vi "Event_Structure.vi"() -> ()   [LabVIEW 2022 SP3]
panel:
  out "Numeric":i32
  out "String":string
  in  "Close Button":bool
  in  "Open Button":bool
  out "Boolean":bool
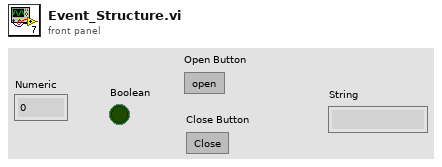
[diagram p1: front panel]
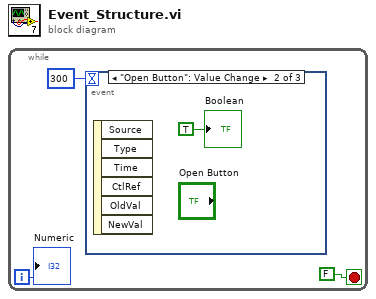
[diagram p0: block diagram]
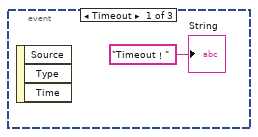
[diagram p2: hidden frame]
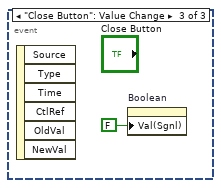
[diagram p3: hidden frame]
diagram:
  n1 = while {
    i -> [w1]
    stop <- FALSE stop-if-true
    n2 = event shown="[1] \"Open Button\": Value Change" {
      selector: _ -> [_ _ _]
      dyn-events: _ -> [_ _ _]
      timeout: 300 -> [_ _ _]
      event Timeout {
        n3 = event-data() -> ()  [unwired: 1 in, 3 out]
        "String" <- "Timeout！" ("String")
      }
      event "Open Button": Value Change {
        n4 = event-data() -> ()  [unwired: 1 in, 6 out]
        "Boolean" <- TRUE ("Boolean")
      }
      event "Close Button": Value Change {
        n5 = event-data() -> ()  [unwired: 1 in, 6 out]
        n6 = property on="Boolean" class="Bool (strict)"("Val(Sgnl)"=FALSE ("Value (Signaling)")) -> ()  [unwired: 2 in, 2 out]
      }
    }
    "Numeric" <- w1
  }
